vi "GetKeyValue_Double.vi"(6 "default":dbl, 9 "key":string, 10 "key value pairs":T1[](array[typedef])) -> (1 "value":dbl, 2 "key value pairs out":T1[](array[typedef]), 5 "found":bool)   [LabVIEW 2017, in "PropertyHelpers.lvlib"]
doc: "Returns the double-precision, floating-point value of a particular key in an array of key-value pairs. Use this VI to get properties from the contents of configuration JSON files that the Global Configuration VIs return."
uses:
  <vilib>/addons/InsightCM/Utilities/PropertyHelpers/PropertyHelpers.lvlib
  <vilib>/addons/InsightCM/MessageBus/Base/controls/KeyValuePair.ctl
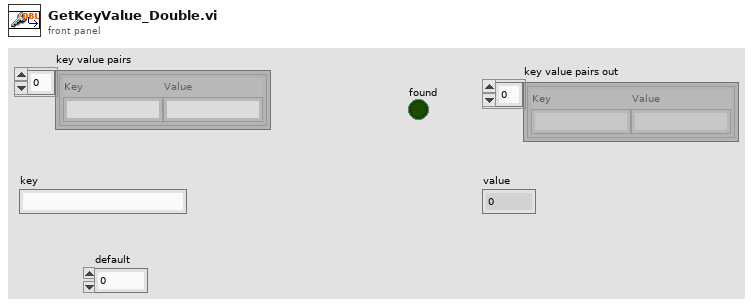
[diagram p1: front panel]
types:
  T1 = typedef "KeyValuePair.ctl" = cluster{"Key":string, "Value":string}
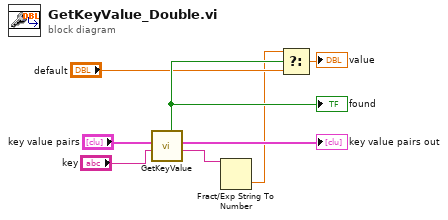
[diagram p0: block diagram]
diagram:
  n1 = call <vilib>:"GetKeyValue.vi"("key"="key", "key value pairs"="key value pairs") -> ("value"=w5:string, "key value pairs out"=→"key value pairs out":T1[], "found"=w4:bool)  [unwired: 7 in]
  "found" <- w4
  n2 = Fract/Exp String To Number(string=w5) -> (number=w2:dbl)  [unwired: 3 in, 1 out]
  n3 = Select(t=w2, s=w4, f="default") -> (s? t:f=→"value":dbl)
